vi "DAQmx Read (Analog 1D Wfm NChan 1Samp).vi"(0 "task/channels in":refnum<k21>, 9 "timeout":dbl=10.0 format="%0.2f", 11 "error in":errorcluster) -> (4 "task out":refnum<k21>, 6 "data":waveform(dbl)[](array[waveform]), 15 "error out":errorcluster)   [LabVIEW 2011]
doc: "Reads a waveform that contains a single sample from each channel in a task that contains one or more analog input channels."
uses:
  nilvaiu.dll
panel:
  # "channel"
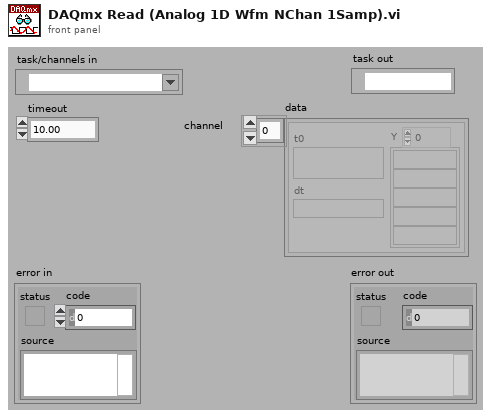
[diagram p1: front panel]
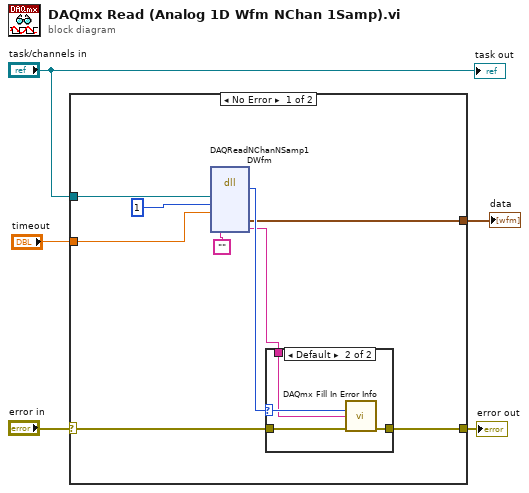
[diagram p0: block diagram]
diagram:
  n1 = case shown="No Error" "error in" {
    selector: "error in" -> [w7 w20]
    tunnel: [w12 w20] -> w4
    tunnel: "task/channels in" -> [w14 _]
    tunnel: [w8 _] -> w2
    tunnel: "timeout" -> [w6 _]
    frame No Error {
      n2 = dll-call lib="nilvaiu.*" fn="DAQReadNChanNSamp1DWfm"("taskID"=w14, "numberOfSamples"=1, "timeout"=w6, "extendedErrorInfo"="") -> (w13:i32, "data"=w8:waveform(dbl)[], "extendedErrorInfo"=w9:string)  [unwired: 5 in, 4 out]
      n3 = case shown="Default" w13 {
        selector: w13 -> [_ w17]
        tunnel: w7 -> [w15 w19]
        tunnel: [w15 w18] -> w12
        tunnel: w9 -> [_ w16]
        frame 0 {
        }
        frame Default {
          n4 = call "DAQmx Fill In Error Info.vi"("status code"=w17, "extended error info"=w16, "error in"=w19) -> ("error out"=w18:errorcluster)  [unwired: 1 in, 11 out]
        }
      }
    }
    frame Error {
    }
  }
  "error out" <- w4
  "data" <- w2
  "task out" <- "task/channels in"
